vi "Reshape Image x8 (Block to Full) (SubVI).vi"(0 "Pixel Data In":u64, 5 "Pixel In Valid?":bool=TRUE, 10 "Block Size":u16=8, 12 "Image Width (/8)":u16=512) -> (14 "Pixel Data Out":u64, 19 "Pixel Out Valid?":bool)   [LabVIEW 2015]
uses:
  Controls (FPGA)/Image Block Readout.ctl
  Controls (FPGA)/Image Block Write.ctl
  <vilib>/rvi/DataTransferAndStorage/Container/Common/niFpgaContainerGetUniqueNameForEmu.vi
  <vilib>/rvi/DataTransferAndStorage/Container/Common/niFpgaContainerSetEmuInfo.vi
  <vilib>/rvi/eio/common/nirviEmuReportErrorAndStop.vi
  <vilib>/rvi/Memory/Memory_Emulation/nirvimemoryFastEmulation.vi
  <vilib>/rvi/Memory/Memory_Emulation/nirvimemoryEmulation.vi
  <vilib>/rvi/Emulation/niFpgaEmulationIsFPGAContextNoSignature.vi
  <vilib>/rvi/Emulation/niFpgaProcessEmulError.vi
  <vilib>/rvi/Emulation/niFpgaSctlEmulationGetInTimedLoop.vi
  <vilib>/rvi/errors/nirviReportUnexpectedCaseInternalError (U32).vi
  <vilib>/rvi/errors/niFpgaSetErrorForExecOnDevCompSimple.vi
  <vilib>/rvi/FIFO/Fifo_Resource/nirvififoEmulationSetSize.vi
  <vilib>/rvi/FIFO/Fifo_Resource/nirviFifoEmulationQueueMgr.vi
  <instcachedir>/0/nirviFifoEmulationQueueMgr_E5CAEC123FF24DC58D834DCA3CDAA9B5.lvgen/nirviFifoEmulationQueueMgr_E5CAEC123FF24DC58D834DCA3CDAA9B5_002.vi
  <vilib>/rvi/FIFO/Fifo_Resource/nirvififoEmulationDetermineInputValidOut.vi
  <vilib>/rvi/FIFO/Fifo_Resource/nirvififoEmulationCreateLock.vi
  <vilib>/rvi/FIFO/Fifo_Resource/nirvififoEmulationObtainLock.vi
  <vilib>/rvi/FIFO/Fifo_Resource/nirvififoEmulationReleaseLock.vi
  <vilib>/rvi/occurrence/nirviWaitOnOccurrenceBase.vi
  <vilib>/rvi/errors/nirviReportUnexpectedCaseInternalError.vi
  <vilib>/Utility/error.llb/Clear Errors.vi
  <vilib>/rvi/LocalResourceManager/LocalResourceManager.xnode
  <vilib>/rvi/DataTransferAndStorage/Container/XNode/niFpgaContainer.xnode
  <vilib>/rvi/FIFO/Fifo_Resource/nirvififoEmulationWrite.vi
  <vilib>/rvi/FIFO/Fifo_Resource/nirvififoEmulationRead.vi
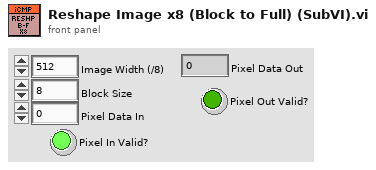
[diagram p1: front panel]
types:
  T1 = typedef "Image Block Readout.ctl" = enum16{"Sync Read", "Read Block Set 1", "Read Block Set 2"}
  T2 = typedef "Image Block Write.ctl" = enum16{"Block 1", "Block 2"}
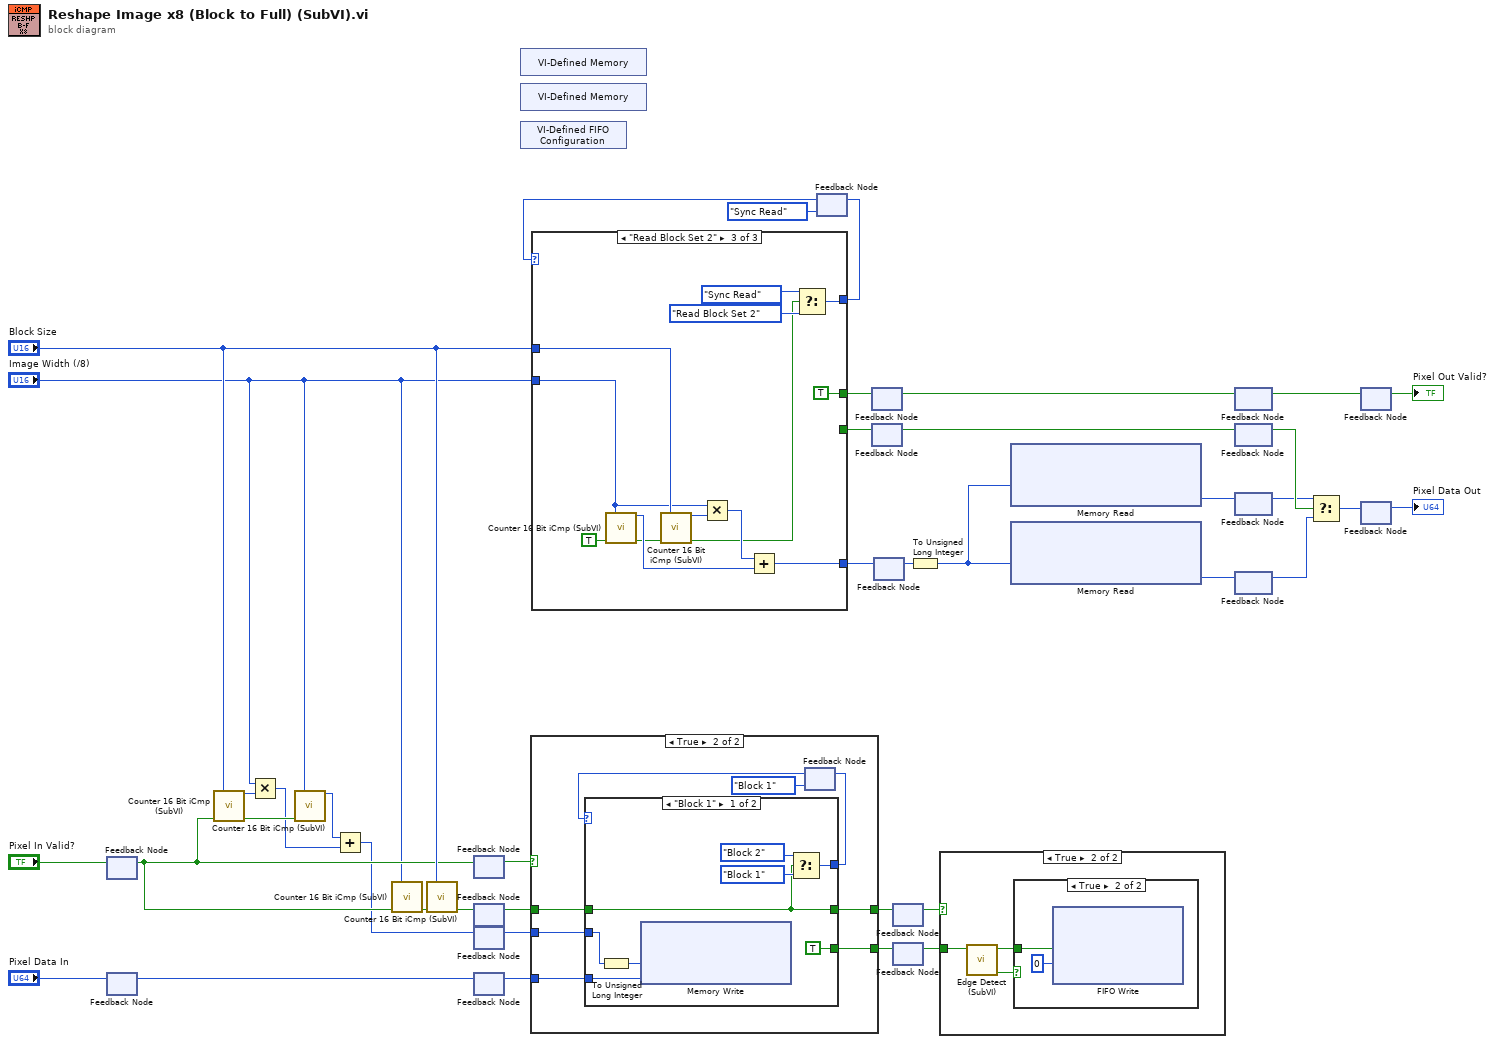
[diagram p0: block diagram]
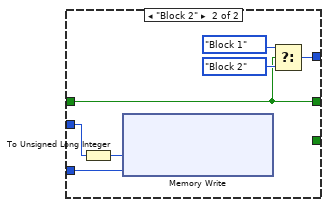
[diagram p5: hidden frame]
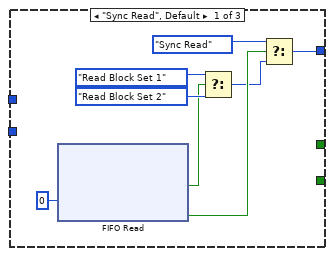
[diagram p6: hidden frame]
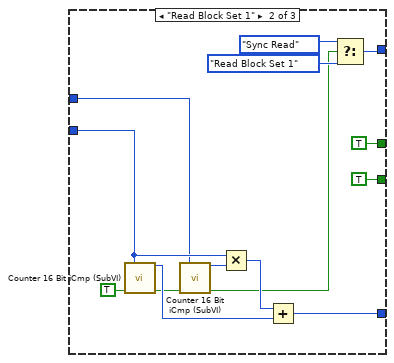
[diagram p7: hidden frame]
diagram:
  n1 = feedback-in #1("Pixel In Valid?") -> ()
  n2 = feedback #1() -> (w8:bool)  [unwired: 1 in]
  n3 = feedback-in #2("Pixel Data In") -> ()
  n4 = feedback #2() -> (w14:u64)  [unwired: 1 in]
  n5 = call "Counter 16 Bit iCmp (SubVI).vi"("Max. Count"="Block Size", "Enable"=w8) -> ("Count"=w7:u16, "Count End?"=w6:bool)  [unwired: 11 in, 1 out]
  n6 = Multiply(x="Image Width (/8)", y=w7) -> (x*y=w4:u16)
  n7 = call "Counter 16 Bit iCmp (SubVI).vi"("Max. Count"="Image Width (/8)", "Enable"=w6) -> ("Count"=w5:u16)  [unwired: 11 in, 2 out]
  n8 = Add(x=w5, y=w4) -> (x+y=w3:u16)
  n9 = call "Counter 16 Bit iCmp (SubVI).vi"("Max. Count"="Image Width (/8)", "Enable"=w8) -> ("Count End?"=w10:bool)  [unwired: 11 in, 2 out]
  n10 = call "Counter 16 Bit iCmp (SubVI).vi"("Max. Count"="Block Size", "Enable"=w10) -> ("Count End?"=w2:bool)  [unwired: 11 in, 2 out]
  n11 = feedback-in #3(w8) -> ()
  n12 = feedback #3() -> (w20:bool)  [unwired: 1 in]
  n13 = feedback-in #4(w2) -> ()
  n14 = feedback #4() -> (w22:bool)  [unwired: 1 in]
  n15 = feedback-in #5(w3) -> ()
  n16 = feedback #5() -> (w21:u16)  [unwired: 1 in]
  n17 = feedback-in #6(w14) -> ()
  n18 = feedback #6() -> (w19:u64)  [unwired: 1 in]
  n19 = xnode "VI-Defined Memory"() -> ()  [unwired: 1 out]
  n20 = xnode "VI-Defined Memory"() -> ()  [unwired: 1 out]
  n21 = xnode "VI-Defined FIFO Configuration"() -> ()  [unwired: 1 out]
  n22 = case shown="True" w20 {
    tunnel: w19 -> [_ w45]
    tunnel: w22 -> [_ w44]
    tunnel: w21 -> [_ w43]
    tunnel: [_ w42] -> w18
    tunnel: [_ w41] -> w17
    frame False {
    }
    frame True {
      n23 = feedback #7(Image_Block_Write."Block 1") -> (w47:T2)
      n24 = case shown="\"Block 1\"" w47 {
        tunnel: w43 -> [w56 w63]
        tunnel: w45 -> [w55 w62]
        tunnel: [w51 w58] -> w48
        tunnel: w44 -> [w49 w57]
        tunnel: [w49 w57] -> w42
        tunnel: [TRUE ("Enable") _] -> w41
        frame "Block 1" {
          n25 = To Unsigned Long Integer(number=w56) -> (unsigned 32bit integer=w54:u32)
          n26 = xnode ("Memory Write")("Address"=w54, "Data"=w55) -> ()  [unwired: 1 in, 1 out]
          n27 = Select(t=Image_Block_Write."Block 2", s=w49, f=Image_Block_Write."Block 1") -> (s? t:f=w51:T2)
        }
        frame "Block 2" {
          n28 = To Unsigned Long Integer(number=w63) -> (unsigned 32bit integer=w61:u32)
          n29 = xnode ("Memory Write")("Address"=w61, "Data"=w62) -> ()  [unwired: 1 in, 1 out]
          n30 = Select(t=Image_Block_Write."Block 1", s=w57, f=Image_Block_Write."Block 2") -> (s? t:f=w58:T2)
        }
      }
      n31 = feedback-in #7(w48) -> ()
    }
  }
  n32 = feedback #8(Image_Block_Readout."Sync Read") -> (w26:T1)
  n33 = case shown="\"Read Block Set 2\"" w26 {
    tunnel: [w70 w83 w96] -> w25
    tunnel: "Block Size" -> [_ w72 w88]
    tunnel: [_ TRUE ("Auto RESET") _] -> w29
    tunnel: [_ TRUE ("Auto RESET") TRUE ("Auto RESET")] -> w28
    tunnel: "Image Width (/8)" -> [_ w73 w87]
    tunnel: [_ w75 w89] -> w11
    frame "Sync Read", Default {
      n34 = xnode ("FIFO Read")("Timeout"=0) -> ("Element"=w65:bool, "Timed Out?"=w68:bool)  [unwired: 1 in, 1 out]
      n35 = Select(t=Image_Block_Readout."Read Block Set 1", s=w65, f=Image_Block_Readout."Read Block Set 2") -> (s? t:f=w64:T1)
      n36 = Select(t=Image_Block_Readout."Sync Read", s=w68, f=w64) -> (s? t:f=w70:T1)
    }
    frame "Read Block Set 1" {
      n37 = call "Counter 16 Bit iCmp (SubVI).vi"("Max. Count"=w73, "Enable"=TRUE) -> ("Count"=w80:u16, "Count End?"=w77:bool)  [unwired: 11 in, 1 out]
      n38 = call "Counter 16 Bit iCmp (SubVI).vi"("Max. Count"=w72, "Enable"=w77) -> ("Count"=w78:u16, "Count End?"=w76:bool)  [unwired: 11 in, 1 out]
      n39 = Multiply(x=w73, y=w78) -> (x*y=w79:u16)
      n40 = Add(x=w79, y=w80) -> (x+y=w75:u16)
      n41 = Select(t=Image_Block_Readout."Sync Read", s=w76, f=Image_Block_Readout."Read Block Set 1") -> (s? t:f=w83:T1)
    }
    frame "Read Block Set 2" {
      n42 = call "Counter 16 Bit iCmp (SubVI).vi"("Max. Count"=w87, "Enable"=TRUE) -> ("Count"=w94:u16, "Count End?"=w91:bool)  [unwired: 11 in, 1 out]
      n43 = call "Counter 16 Bit iCmp (SubVI).vi"("Max. Count"=w88, "Enable"=w91) -> ("Count"=w92:u16, "Count End?"=w86:bool)  [unwired: 11 in, 1 out]
      n44 = Multiply(x=w87, y=w92) -> (x*y=w93:u16)
      n45 = Add(x=w93, y=w94) -> (x+y=w89:u16)
      n46 = Select(t=Image_Block_Readout."Sync Read", s=w86, f=Image_Block_Readout."Read Block Set 2") -> (s? t:f=w96:T1)
    }
  }
  n47 = feedback-in #8(w25) -> ()
  n48 = feedback #9() -> (w30:bool)  [unwired: 1 in]
  n49 = feedback-in #9(w28) -> ()
  n50 = feedback #10() -> (w31:bool)  [unwired: 1 in]
  n51 = feedback-in #10(w29) -> ()
  n52 = feedback #11() -> (w32:u16)  [unwired: 1 in]
  n53 = feedback-in #11(w11) -> ()
  n54 = feedback-in #12(w18) -> ()
  n55 = feedback #12() -> (w16:bool)  [unwired: 1 in]
  n56 = feedback-in #13(w17) -> ()
  n57 = feedback #13() -> (w15:bool)  [unwired: 1 in]
  n58 = To Unsigned Long Integer(number=w32) -> (unsigned 32bit integer=w33:u32)
  n59 = case shown="True" w16 {
    tunnel: w15 -> [_ w99]
    frame False {
    }
    frame True {
      n60 = call "Edge Detect (SubVI).vi"("TTL In"=w99) -> ("Edge?"=w101:bool, "Rising Edge"=w100:bool)  [unwired: 8 in, 1 out]
      n61 = case shown="True" w101 {
        tunnel: w100 -> [_ w102]
        frame False {
        }
        frame True {
          n62 = xnode ("FIFO Write")("Element"=w102, "Timeout"=0) -> ()  [unwired: 1 in, 2 out]
        }
      }
    }
  }
  n63 = xnode ("Memory Read")("Address"=w33) -> ("Data"=w35:u64)  [unwired: 1 in, 1 out]
  n64 = xnode ("Memory Read")("Address"=w33) -> ("Data"=w34:u64)  [unwired: 1 in, 1 out]
  n65 = feedback #14() -> (w36:bool)  [unwired: 1 in]
  n66 = feedback-in #14(w30) -> ()
  n67 = feedback #15() -> (w39:bool)  [unwired: 1 in]
  n68 = feedback-in #15(w31) -> ()
  n69 = feedback #16() -> (w37:u64)  [unwired: 1 in]
  n70 = feedback-in #16(w35) -> ()
  n71 = feedback #17() -> (w38:u64)  [unwired: 1 in]
  n72 = feedback-in #17(w34) -> ()
  n73 = Select(t=w37, s=w39, f=w38) -> (s? t:f=w40:u64)
  n74 = feedback-in #18(w36) -> ()
  n75 = feedback #18() -> (→"Pixel Out Valid?":bool)  [unwired: 1 in]
  n76 = feedback-in #19(w40) -> ()
  n77 = feedback #19() -> (→"Pixel Data Out":u64)  [unwired: 1 in]
